vi "update-table.vi"(4 "error in (no error)":errorcluster, 6 "contents":T1(array[cluster]), 7 "Table ref in":refnum<vi>) -> (0 "error out":errorcluster, 3 "Table ref out":refnum<vi>)   [LabVIEW 2016]
panel:
  out "content update":string[][](array[string])
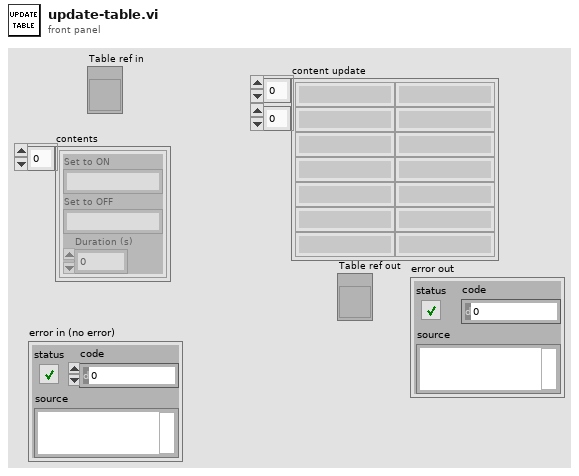
[diagram p1: front panel]
types:
  T1 = cluster{"Set to ON":string, "Set to OFF":string, "Duration (s)":i32}[]
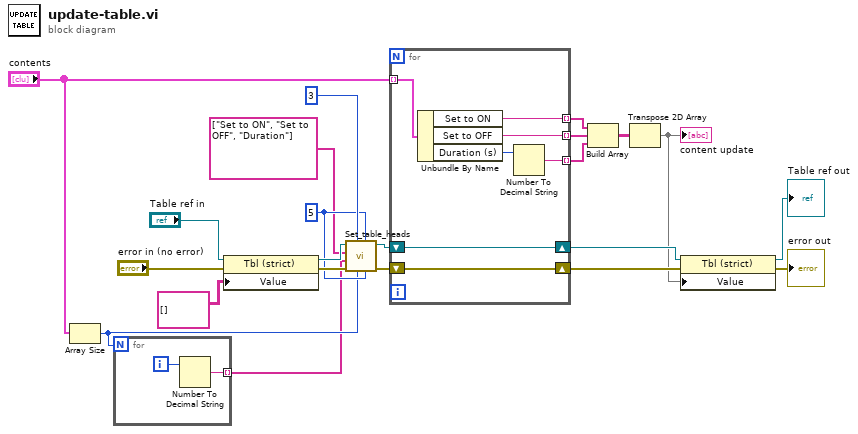
[diagram p0: block diagram]
diagram:
  w16 = i16 5 ("Columm additional width")
  n1 = Array Size(array="contents") -> (size(s)=w14:i32)
  n2 = for {
    N: w14 -> [_]
    tunnel: [w23] -> w13 mode=indexing
    i -> [w24]
    n3 = Number To Decimal String(number=w24) -> (decimal integer string=w23:string)  [unwired: 1 in]
  }
  n4 = property on="Property Node" class="Tbl (strict)"(reference="Table ref in", error in="error in (no error)", "Value"=string[][] [] ("Table Control")) -> (reference out=w19:refnum<vi>, error out=w18:errorcluster)
  n5 = call "Set_table_heads.vi"("additional row width"=w16, "Columm additional width"=w16, "Number of rows"=w14, "Number of columns"=u32 3, "error in (no error)"=w18, "Row texts"=w13, "Column texts"=string[] ["Set to ON", "Set to OFF", "Duration"], "Table ref in"=w19) -> ("error out"=w11:errorcluster, "Table ref out"=w12:refnum<vi>)  [unwired: 2 in]
  n6 = for {
    shift-right: [w26] -> w4
    shift-left: w11 -> [w26]
    tunnel: "contents" -> [w31] mode=indexing
    tunnel: [w29] -> w9 mode=indexing
    tunnel: [w28] -> w8 mode=indexing
    tunnel: [w27] -> w7 mode=indexing
    shift-right: [w25] -> w5
    shift-left: w12 -> [w25]
    n7 = Unbundle By Name(w31) -> ("Set to ON"=w29:string, "Set to OFF"=w28:string, "Duration (s)"=w30:i32)
    n8 = Number To Decimal String(number=w30) -> (decimal integer string=w27:string)  [unwired: 1 in]
  }
  n9 = Build Array(w9, w8, w7) -> (w6:string[][])
  n10 = Transpose 2D Array(2D array=w6) -> (transposed array=w3:string[][])
  "content update" <- w3
  n11 = property on="Property Node" class="Tbl (strict)"(reference=w5, error in=w4, "Value"=w3) -> (reference out=→"Table ref out":refnum<vi>, error out=→"error out":errorcluster)
